vi "DemoCPUUsage.vi"() -> ()   [LabVIEW 2010, in "kevLib2010.lvlib"]
uses:
  kevLib2010.lvlib
  SubVIs/esm_Set Target CPU Monitoring__NATIONAL INSTRUMENTS.vi
  SubVIs/esm_Get Target CPU Usage__NATIONAL INSTRUMENTS.vi
  SubVIs/InterpCPUUsage.vi
panel:
  out "error out":errorcluster
  in  "faster?":bool
  out "UsageNormal":dbl
  out "UsageTimeCritical":dbl
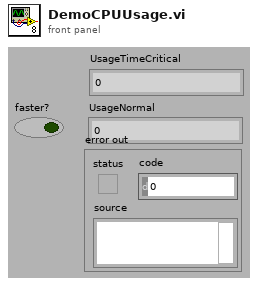
[diagram p1: front panel]
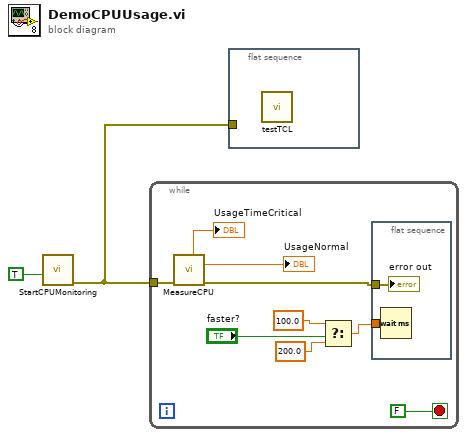
[diagram p0: block diagram]
diagram:
  n1 = call "StartCPUMonitoring.vi"("CPU Monitoring On (T)"=TRUE ("CPU Monitoring On")) -> ("error out"=w1:errorcluster)  [unwired: 10 in]
  n2 = while {
    tunnel: w1 -> [w6]
    stop <- FALSE stop-if-true
    n3 = call "MeasureCPU.vi"("error in (no error)"=w6) -> ("error out"=w8:errorcluster, "Normal Priority"=→"UsageNormal":dbl, "Time Critical"=→"UsageTimeCritical":dbl)  [unwired: 6 in, 2 out]
    n4 = Select(t=100.0, s="faster?", f=200.0 ("t")) -> (s? t:f=w9:dbl)
    n5 = flat-sequence {
      tunnel: w9 -> [w13]
      tunnel: w8 -> [w12]
      frame #0 {
        n6 = Wait (ms)(milliseconds to wait=w13) -> ()  [unwired: 1 out]
        "error out" <- w12
      }
    }
  }
  n7 = flat-sequence {
    tunnel: w1 -> [_]
    frame #0 {
      n8 = call "testTCL.vi"() -> ()  [unwired: 1 in]
    }
  }
